vi "ECG_bruité_filté.vi"() -> ()   [LabVIEW 2018]
uses:
  <vilib>/measure/maspectr.llb/FFT Spectrum (Mag-Phase) for 1 Chan.vi
  <vilib>/Analysis/3filter.llb/Butterworth Filter (DBL).vi
  <vilib>/Analysis/NI_AALBase.lvlib
  <vilib>/measure/NI_MAPro.lvlib
panel:
  in  "Numeric Control":dbl=7.0
  in  "nb des périodes 4":dbl=2.0
  in  "nb des périodes 3":dbl=2.0
  in  "nb des périodes":dbl=2.0
  out "Waveform Graph 8":cluster{"f0":dbl, "df":dbl, "magnitude":dbl[]}(graph)
  out "Waveform Graph 7":waveform(dbl)(graph)
  out "Waveform Graph 6":cluster{"f0":dbl, "df":dbl, "magnitude":dbl[]}(graph)
  out "Waveform Graph 5":cluster{"f0":dbl, "df":dbl, "magnitude":dbl[]}(graph)
  out "Waveform Graph 3":waveform(dbl)(graph)
  out "Waveform Graph":waveform(dbl)(graph)
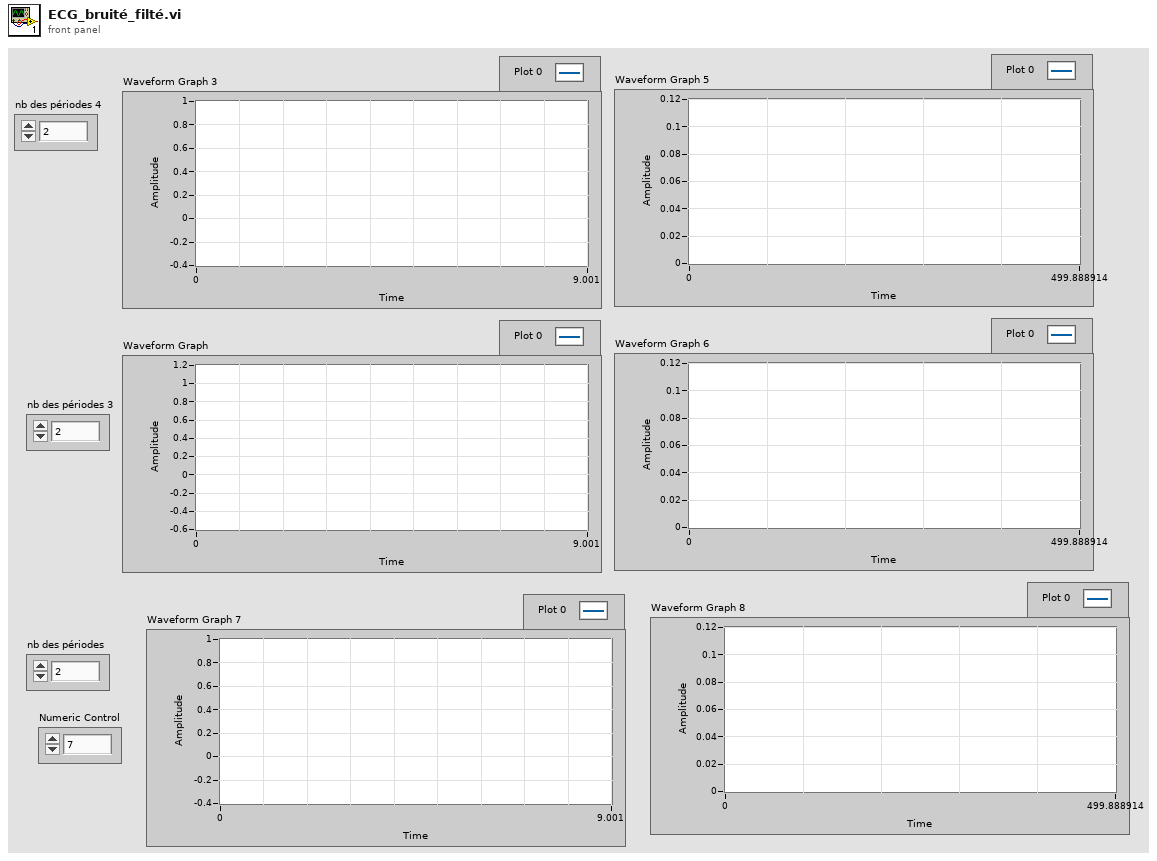
[diagram p1: front panel]
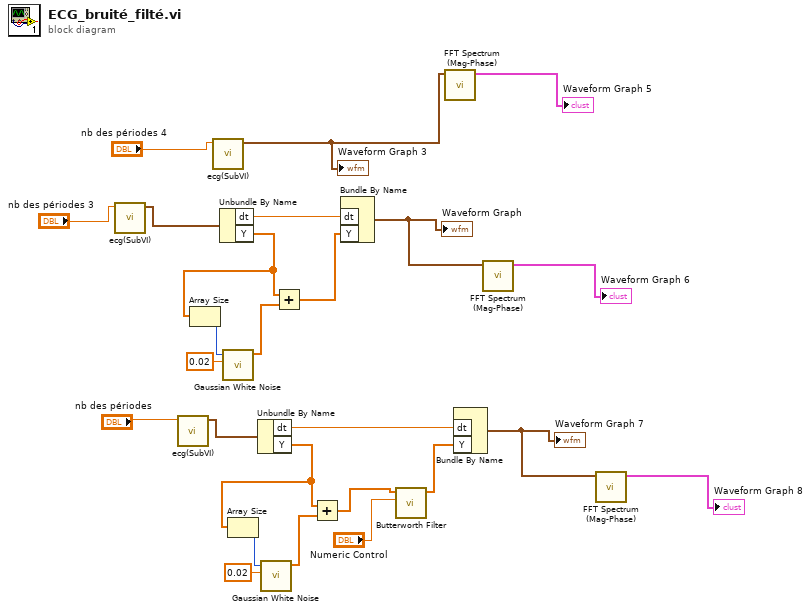
[diagram p0: block diagram]
diagram:
  n1 = call "ecg(SubVI).vi"("nb de période"="nb des périodes 3") -> ("signal out"=w5:waveform(dbl))  [unwired: 10 in]
  n2 = call "ecg(SubVI).vi"("nb de période"="nb des périodes") -> ("signal out"=w11:waveform(dbl))  [unwired: 10 in]
  n3 = call "ecg(SubVI).vi"("nb de période"="nb des périodes 4") -> ("signal out"=w1:waveform(dbl))  [unwired: 10 in]
  "Waveform Graph 3" <- w1
  n4 = Unbundle By Name(w5) -> ("dt"=w12:dbl, "Y"=w6:dbl[])
  n5 = Array Size(array=w6) -> (size(s)=w23:i32)
  n6 = call <vilib>:"Gaussian White Noise.vi"("standard deviation"=0.02, "samples"=w23) -> ("Gaussian noise pattern"=w25:dbl[])  [unwired: 8 in, 1 out]
  n7 = Unbundle By Name(w11) -> ("dt"=w13:dbl, "Y"=w4:dbl[])
  n8 = Array Size(array=w4) -> (size(s)=w18:i32)
  n9 = call <vilib>:"Gaussian White Noise.vi"("standard deviation"=0.02, "samples"=w18) -> ("Gaussian noise pattern"=w19:dbl[])  [unwired: 8 in, 1 out]
  n10 = Add(x=w6, y=w25) -> (x+y=w24:dbl[])
  n11 = Add(x=w4, y=w19) -> (x+y=w15:dbl[])
  n12 = Bundle By Name("dt"=w12, "Y"=w24) -> (w20:waveform(dbl))  [unwired: 1 in]
  "Waveform Graph" <- w20
  n13 = call-poly <vilib>:"Butterworth Filter.vi"("sampling freq: fs"="Numeric Control", "X"=w15) -> ("Filtered X"=w14:dbl[])  [unwired: 6 in, 1 out]
  n14 = call-poly <vilib>:"FFT Spectrum (Mag-Phase).vi"("time signal"=w1) -> ("magnitude"=→"Waveform Graph 5":cluster{"f0":dbl, "df":dbl, "magnitude":dbl[]})  [unwired: 6 in, 4 out]
  n15 = Bundle By Name("dt"=w13, "Y"=w14) -> (w16:waveform(dbl))  [unwired: 1 in]
  "Waveform Graph 7" <- w16
  n16 = call-poly <vilib>:"FFT Spectrum (Mag-Phase).vi"("time signal"=w20) -> ("magnitude"=→"Waveform Graph 6":cluster{"f0":dbl, "df":dbl, "magnitude":dbl[]})  [unwired: 6 in, 4 out]
  n17 = call-poly <vilib>:"FFT Spectrum (Mag-Phase).vi"("time signal"=w16) -> ("magnitude"=→"Waveform Graph 8":cluster{"f0":dbl, "df":dbl, "magnitude":dbl[]})  [unwired: 6 in, 4 out]
